vi "DBM Delete Data.vi"(5 "Query info":T1, 7 "데이터":T4, 8 "에러 입력":errorcluster caption="에러 입력(에러 없음)", 10 "추가?":bool, 11 "참조 번호 입력":T2) -> (0 "에러 출력":errorcluster, 2 "COMMAND":T3, 3 "참조 번호 출력":T2)   [LabVIEW 2020]
uses:
  <vilib>/addons/database/Connection.llb/Conn ObjectReference.ctl
  Controls/Clst_DBM data.ctl
  Controls/Cmd_Write Query.ctl
  Controls/Clst_Query Info.ctl
  <vilib>/addons/database/NI_Database_API.lvlib
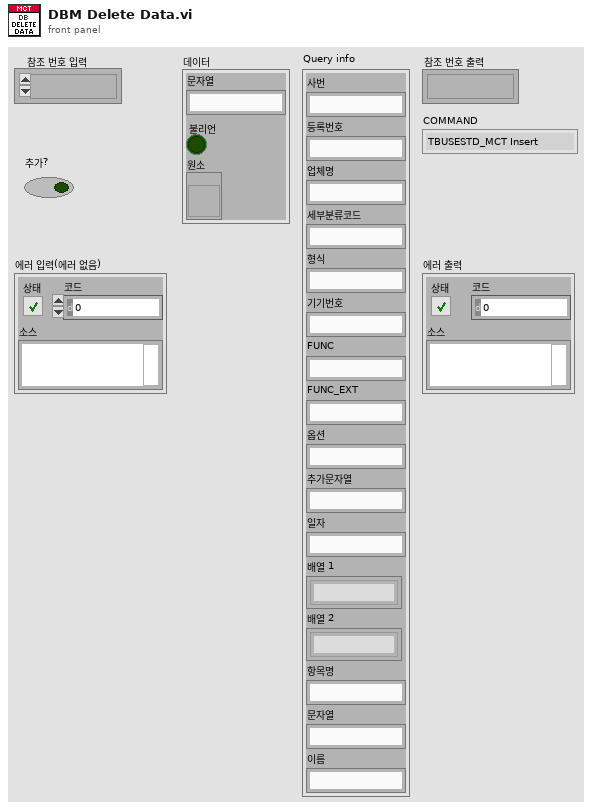
[diagram p1: front panel]
types:
  T1 = typedef "Clst_Query Info.ctl" = cluster{"사번":string, "등록번호":string, "업체명":string, "세부분류코드":string, "형식":string, "기기번호":string, "FUNC":string, "FUNC_EXT":string, "옵션":string, "추가문자열":string, "일자":string, "배열 1":string[], "배열 2":string[], "항목명":string, "문자열":string, "이름":string}
  T2 = typedef "NI_Database_API.lvlib/Conn ObjectReference.ctl" = refnum<k1>
  T3 = typedef "Cmd_Write Query.ctl" = enum16{"TBUSESTD_MCT Insert", "TBUSESTD_MCT Delete", "TBCALSTD_MCT_TEMP Insert", "TBCALSTD_MCT_TEMP Delete", "TBCALSTD_MCT Insert", "TBCALSTD_MCT Delete", "TBCALSTD_MCT_BACK Insert", "TBCALSTD_MCT_BACK Delete", "TBCALPROC_MCT Insert", "TBCALPROC_MCT Delete", "TBCALPROC_MCT_TEMP Insert", "TBCALPROC_MCT_TEMP Delete", "TBCALCMC_MCT Insert", "TBCALCMC_MCT Delete", "TBCALFUNC_MCT Insert", "TBCALFUNC_MCT Delete", "TBCALNAME_MCT Insert", "TBCALNAME_MCT Delete", "TBSTDNAME_MCT Insert", "TBSTDNAME_MCT Delete", "TBCALSPEC_MCT Insert", "TBCALSPEC_MCT Delete", "TBCALSTD_MCT NOTUSE update", "TBCALSPEC_MCT update", "TBMCTVERMAN update"}
  T4 = typedef "Clst_DBM data.ctl" = cluster{"문자열":string, "불리언":bool, "원소":refnum<vi>}
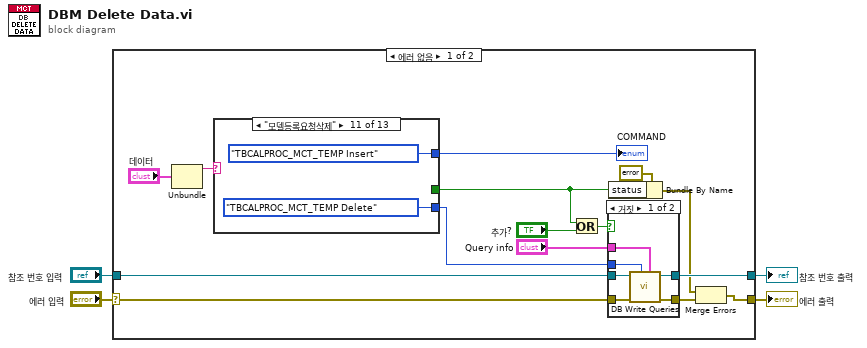
[diagram p0: block diagram]
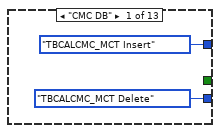
[diagram p3: hidden frame]
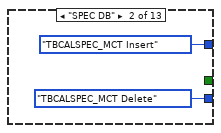
[diagram p4: hidden frame]
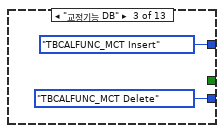
[diagram p5: hidden frame]
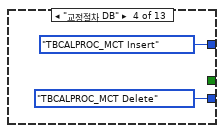
[diagram p6: hidden frame]
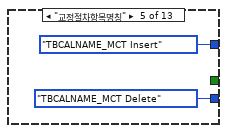
[diagram p7: hidden frame]
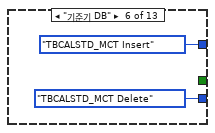
[diagram p8: hidden frame]
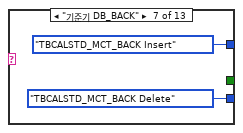
[diagram p9: hidden frame]
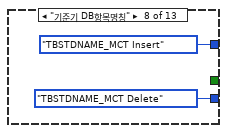
[diagram p10: hidden frame]
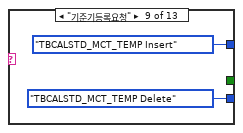
[diagram p11: hidden frame]
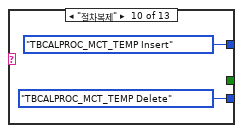
[diagram p12: hidden frame]
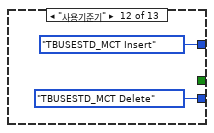
[diagram p13: hidden frame]
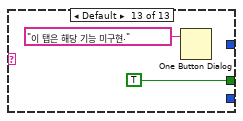
[diagram p14: hidden frame]
diagram:
  n1 = case shown="에러 없음" "에러 입력" {
    selector: "에러 입력" -> [w15 w55]
    tunnel: [w8 w55] -> w4
    tunnel: [w19 w54] -> w3
    tunnel: "참조 번호 입력" -> [w16 w54]
    frame No Error {
      n2 = Unbundle("데이터") -> ("문자열"=w10:string)  [unwired: 2 out]
      n3 = case shown="\"모델등록요청삭제\"" w10 {
        tunnel: [_ _ _ _ _ _ _ _ _ _ _ _ TRUE] -> w6
        tunnel: [Cmd_Write_Query."TBCALCMC_MCT Delete" ("COMMAND") Cmd_Write_Query."TBCALSPEC_MCT Delete" ("COMMAND") Cmd_Write_Query."TBCALFUNC_MCT Delete" ("COMMAND") Cmd_Write_Query."TBCALPROC_MCT Delete" ("COMMAND") Cmd_Write_Query."TBCALNAME_MCT Delete" ("COMMAND") Cmd_Write_Query."TBCALSTD_MCT Delete" ("COMMAND") Cmd_Write_Query."TBCALSTD_MCT_BACK Delete" ("COMMAND") Cmd_Write_Query."TBSTDNAME_MCT Delete" ("COMMAND") Cmd_Write_Query."TBCALSTD_MCT_TEMP Delete" ("COMMAND") Cmd_Write_Query."TBCALPROC_MCT_TEMP Delete" ("COMMAND") Cmd_Write_Query."TBCALPROC_MCT_TEMP Delete" ("COMMAND") Cmd_Write_Query."TBUSESTD_MCT Delete" ("COMMAND") _] -> w18
        tunnel: [Cmd_Write_Query."TBCALCMC_MCT Insert" ("COMMAND") Cmd_Write_Query."TBCALSPEC_MCT Insert" ("COMMAND") Cmd_Write_Query."TBCALFUNC_MCT Insert" ("COMMAND") Cmd_Write_Query."TBCALPROC_MCT Insert" ("COMMAND") Cmd_Write_Query."TBCALNAME_MCT Insert" ("COMMAND") Cmd_Write_Query."TBCALSTD_MCT Insert" ("COMMAND") Cmd_Write_Query."TBCALSTD_MCT_BACK Insert" ("COMMAND") Cmd_Write_Query."TBSTDNAME_MCT Insert" ("COMMAND") Cmd_Write_Query."TBCALSTD_MCT_TEMP Insert" ("COMMAND") Cmd_Write_Query."TBCALPROC_MCT_TEMP Insert" ("COMMAND") Cmd_Write_Query."TBCALPROC_MCT_TEMP Insert" ("COMMAND") Cmd_Write_Query."TBUSESTD_MCT Insert" ("COMMAND") _] -> w17
        frame "CMC DB" {
        }
        frame "SPEC DB" {
        }
        frame "교정기능 DB" {
        }
        frame "교정절차 DB" {
        }
        frame "교정절차항목명칭" {
        }
        frame "기준기 DB" {
        }
        frame "기준기 DB_BACK" {
        }
        frame "기준기 DB항목명칭" {
        }
        frame "기준기등록요청" {
        }
        frame "절차복제" {
        }
        frame "모델등록요청삭제" {
        }
        frame "사용기준기" {
        }
        frame Default {
          n4 = One Button Dialog(message="이 탭은 해당 기능 미구현." ("메시지")) -> ()  [unwired: 1 in, 1 out]
        }
      }
      "COMMAND" <- w17
      n5 = Or(x=w6, y="추가?") -> (x .or. y?=w14:bool)
      n6 = case shown="거짓" w14 {
        tunnel: [w25 w26] -> w9
        tunnel: [w24 w27] -> w19
        tunnel: "Query info" -> [w23 _]
        tunnel: w18 -> [w22 _]
        tunnel: w16 -> [w21 w27]
        tunnel: w15 -> [w20 w26]
        frame False {
          n7 = call "DB Write Queries.vi"("Query info"=w23, "COMMAND"=w22, "에러 입력(에러 없음)"=w20, "참조 번호 입력"=w21) -> ("에러 출력"=w25:errorcluster, "참조 번호 출력"=w24:T2)  [unwired: 6 in]
        }
        frame True {
        }
      }
      n8 = Bundle By Name(cluster=errorcluster {"status"=FALSE, "code"=0, "source"=""} ("에러 입력"), "status"=w6) -> (w5:errorcluster)
      n9 = Merge Errors(w5, w9) -> (w8:errorcluster)
    }
    frame Error {
    }
  }
  "에러 출력" <- w4
  "참조 번호 출력" <- w3
